vi "SW_Init_Array_of_Conditions_2.vi"(2 "Error In":errorcluster) -> (0 "Error Out":errorcluster, 1 "Array of conditions":T1)   [LabVIEW 2018, in "Tracker.lvlib"]
uses:
  Tracker.lvlib
  Classes/Reward_Condition/Controls/RC_Array_of_Conditions.ctl
  Classes/Reward_Condition/Reward_Condition.lvclass
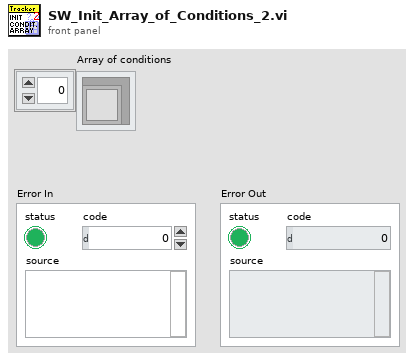
[diagram p1: front panel]
types:
  T1 = typedef "Tracker.lvlib/Reward_Condition.lvclass/RC_Array_of_Conditions.ctl" = refnum<class "Reward_Condition.lvclass">[]
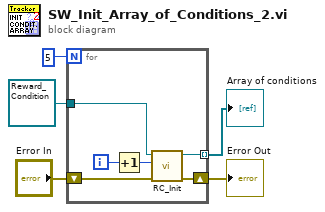
[diagram p0: block diagram]
diagram:
  n1 = for {
    N: 5 -> [_]
    tunnel: refnum<class "Reward_Condition.lvclass"> refnum ("Tracker.lvlib:Reward_Condition.lvclass") -> [w11]
    shift-right: [w7] -> w1
    shift-left: "Error In" -> [w8]
    tunnel: [w6] -> w3 mode=indexing
    i -> [w10]
    n2 = Increment(x=w10) -> (x+1=w9:i32)
    n3 = call "RC_Init.vi"("error in (no error)"=w8, "Condition #"=w9, "Reward_Condition in"=w11) -> ("error out"=w7:errorcluster, "Reward_Condition out"=w6:refnum<class "Reward_Condition.lvclass">)  [unwired: 7 in]
  }
  "Array of conditions" <- w3
  "Error Out" <- w1
